vi "LWXPS_PositionerSGammaParametersSet.vi"(0 "Positioner Name":string, 1 "XPS Reference IN":refnum<k24>, 5 "Motion velocity":dbl, 7 "Motion acceleration":dbl, 9 "Minimum jerk time":dbl, 11 "Maximum jerk time":dbl, 12 "LabVIEW error IN":errorcluster) -> (4 "XPS Reference OUT":refnum<k24>, 6 "Returned error code":i32, 8 "XPS Error String":string, 15 "LabVIEW error OUT":errorcluster)   [LabVIEW 2014]
uses:
  D:/XPSQ8_LabView_Library/Development/Source/Dll/Newport.XPS.CommandInterface.dll
  Dll/Newport.XPS.CommandInterface.dll
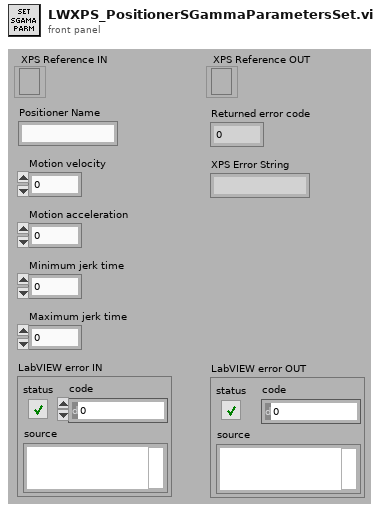
[diagram p1: front panel]
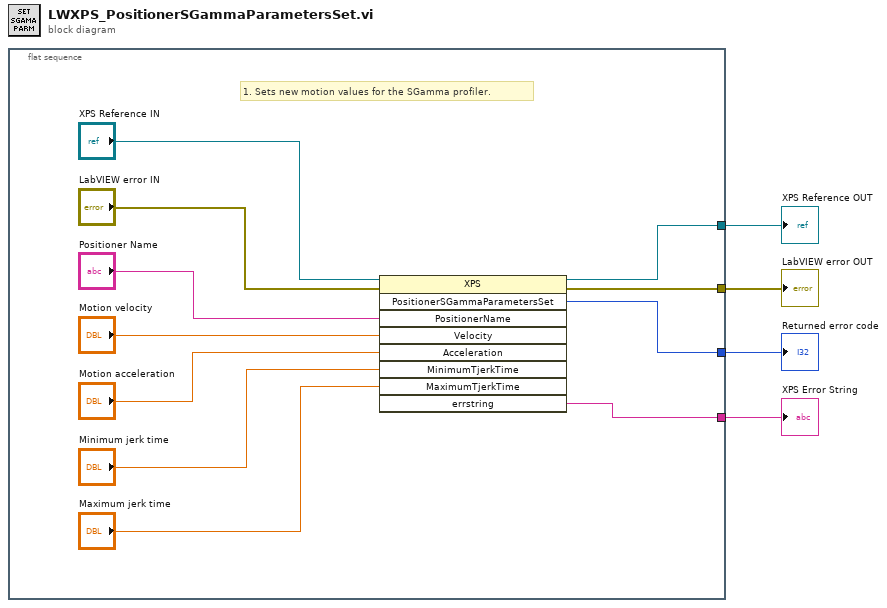
[diagram p0: block diagram]
diagram:
  n1 = flat-sequence {
    tunnel: [w11] -> w4
    tunnel: [w10] -> w3
    tunnel: [w12] -> w2
    tunnel: [w8] -> w1
    frame #0 {
      # "1. Sets new motion values for the SGamma profiler."
      n2 = invoke class="XPS" method="PositionerSGammaParametersSet"(reference="XPS Reference IN", error in="LabVIEW error IN", "PositionerName"="Positioner Name", "Velocity"="Motion velocity", "Acceleration"="Motion acceleration", "MinimumTjerkTime"="Minimum jerk time", "MaximumTjerkTime"="Maximum jerk time") -> (reference out=w11:refnum<k24>, error out=w10:errorcluster, "PositionerSGammaParametersSet"=w12:i32, "errstring"=w8:string)  [unwired: 2 in, 5 out]
    }
  }
  "XPS Error String" <- w1
  "XPS Reference OUT" <- w4
  "LabVIEW error OUT" <- w3
  "Returned error code" <- w2
